vi "_setVariant.vi"(8 "error in (no error)":errorcluster, 9 "value":variant, 10 "name":string, 11 "DB Ref":T1) -> (0 "error in (no error) (dup)":errorcluster, 3 "DB Ref (dup)":T1, 4 "created?":bool)   [LabVIEW 2017, in "TagDB(dev).lvlib"]
uses:
  TagDB(dev).lvlib
  tagDB_Def.ctl
  <userlib>/_OpenG.lib/string/string.llb/Trim Whitespace (String)__ogtk.vi
  Error/_Build Error Cluster.vi
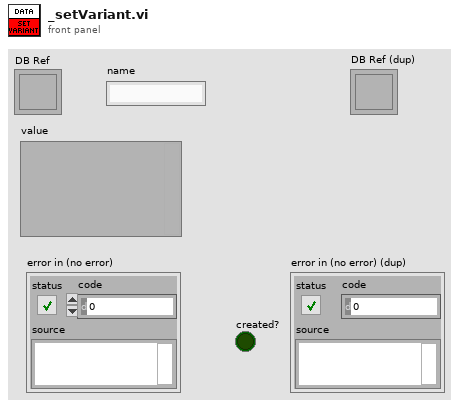
[diagram p1: front panel]
types:
  T1 = typedef "TagDB(dev).lvlib/tagDB_Def.ctl" = refnum<k1>
  T2 = typedef "TagDB(dev).lvlib/_DEF-DATA.ctl" = cluster{"data hashmap":variant, "DataChangeFlag":i64, "ItemChangeFlag":i64, "name":string, "Tag Adding Lock?":bool}
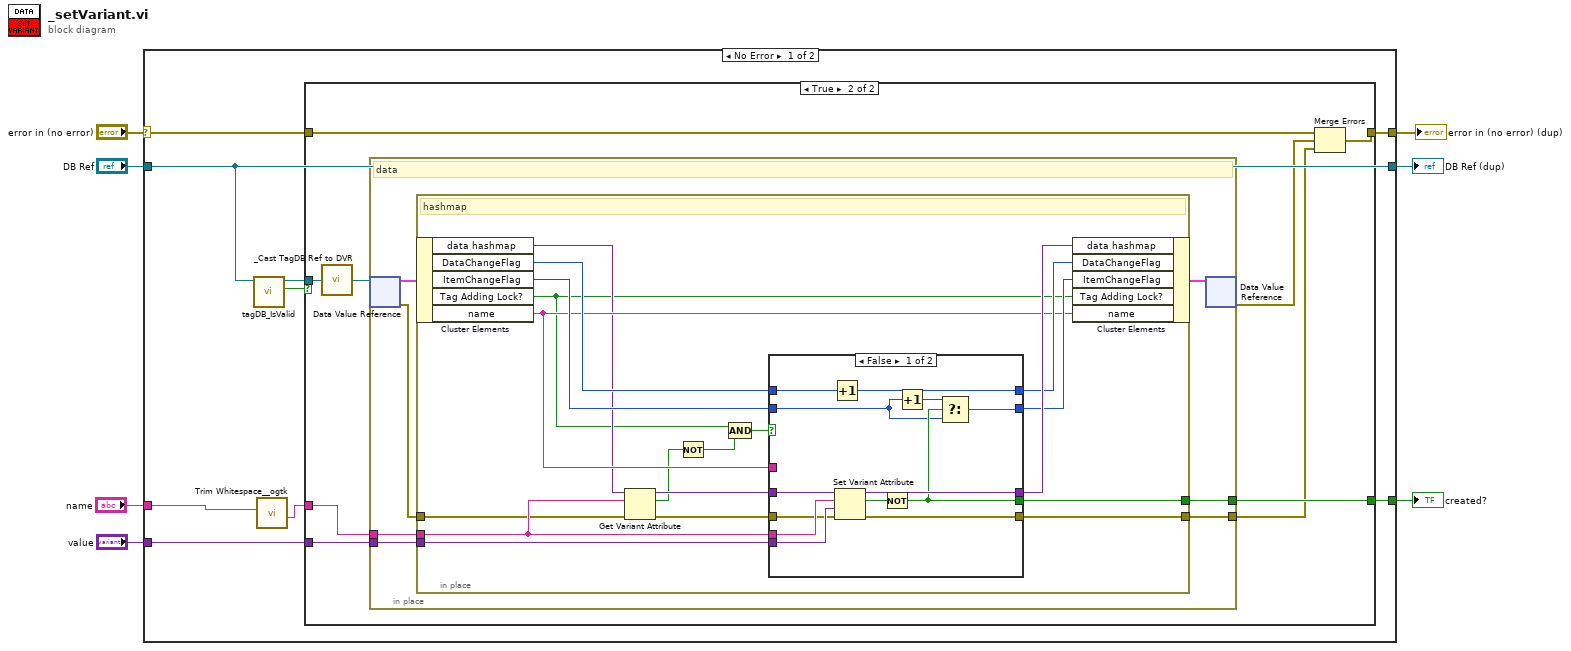
[diagram p0: block diagram]
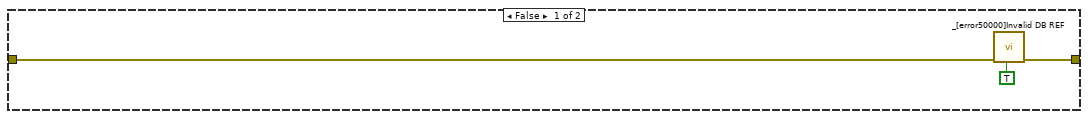
[diagram p2: hidden frame]
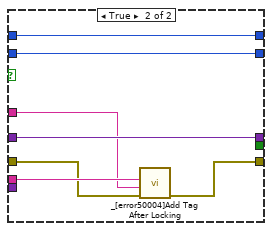
[diagram p3: hidden frame]
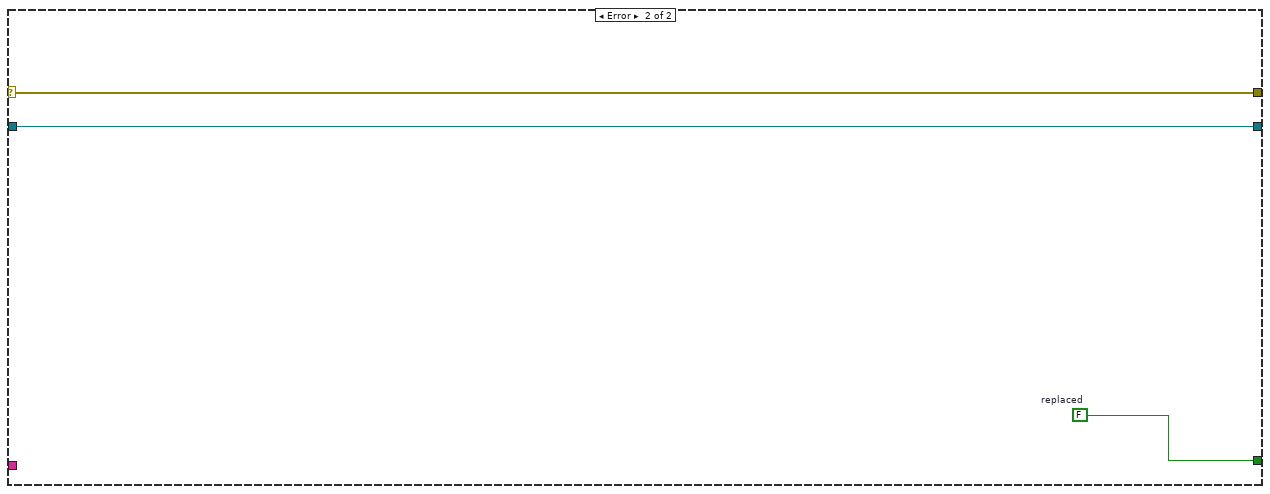
[diagram p4: hidden frame]
diagram:
  n1 = case shown="No Error" "error in (no error)" {
    selector: "error in (no error)" -> [w9 w75]
    tunnel: [w11 w76] -> w7
    tunnel: "DB Ref" -> [w11 w76]
    tunnel: [w15 w75] -> w4
    tunnel: [w16 w74] -> w3
    tunnel: "name" -> [w14 _]
    tunnel: "value" -> [w12 _]
    frame No Error {
      n2 = call "tagDB_IsValid.vi"("DB Ref in"=w11) -> ("valid?"=w8:bool, "DB Ref out"=w10:T1)  [unwired: 8 in, 1 out]
      n3 = call-poly <userlib>:"Trim Whitespace__ogtk.vi"("String in"=w14) -> ("String out"=w13:string)  [unwired: 6 in]
      n4 = case shown="True" w8 {
        tunnel: [_ w28] -> w16
        tunnel: [w18 w27] -> w15
        tunnel: w13 -> [_ w26]
        tunnel: w12 -> [_ w25]
        tunnel: w10 -> [_ w22]
        tunnel: w9 -> [w19 w21]
        frame False {
          n5 = call "_[error50000]Invalid DB REF.vi"("Force Gen?"=TRUE, "error in (no error)"=w19) -> ("error out"=w18:errorcluster)  [unwired: 9 in]
        }
        frame True {
          n6 = call "_Cast TagDB Ref to DVR.vi"("TagDB"=w22) -> ("DVR"=w23:refnum<data-value>)  [unwired: 4 in]
          n7 = in-place {
            in-place-border: [w33] -> w28
            in-place-border: w26 -> [w32]
            in-place-border: w25 -> [w31]
            in-place-border: [w30] -> w24
            # "data"
            n8 = in-place-dvr #1(w23) -> (w35:T2, w29:errorcluster)
            n9 = in-place {
              in-place-border: [w48] -> w33
              in-place-border: w32 -> [w38]
              in-place-border: w31 -> [w52]
              in-place-border: [w49] -> w30
              in-place-border: w29 -> [w36]
              # "hashmap"
              n10 = in-place-cluster #2(w35) -> ("data hashmap"=w44:variant, "DataChangeFlag"=w51:i64, "ItemChangeFlag"=w46:i64, "Tag Adding Lock?"=w40:bool, "name"=w45:string)
              n11 = Get Variant Attribute(Variant=w44, name=w38, error in=w36) -> (duplicate Variant=w43:variant, found=w41:bool, error out=w42:errorcluster)  [unwired: 1 in, 1 out]
              n12 = Not(x=w41) -> (.not. x?=w37:bool)
              n13 = Compound Arithmetic op=AND(w40, w37) -> (w39:bool)
              n14 = case shown="False" w39 {
                tunnel: w43 -> [w66 w73]
                tunnel: [w65 w73] -> w53
                tunnel: w38 -> [w63 w69]
                tunnel: w52 -> [w62 _]
                tunnel: w51 -> [w61 w72]
                tunnel: [w60 w72] -> w50
                tunnel: [w59 w70] -> w49
                tunnel: [w58 _] -> w48
                tunnel: [w57 w71] -> w47
                tunnel: w46 -> [w55 w71]
                tunnel: w45 -> [_ w68]
                tunnel: w42 -> [w54 w67]
                frame False {
                  n15 = Increment(x=w61) -> (x+1=w60:i64)
                  n16 = Set Variant Attribute(Variant=w66, name=w63, value=w62, error in=w54) -> (Variant out=w65:variant, replaced=w64:bool, error out=w59:errorcluster)
                  n17 = Not(x=w64) -> (.not. x?=w58:bool)
                  n18 = Increment(x=w55) -> (x+1=w56:i64)
                  n19 = Select(t=w56, s=w58, f=w55) -> (s? t:f=w57:i64)
                }
                frame True {
                  n20 = call "_[error50004]Add Tag After Locking.vi"("error in (no error)"=w67, "db name"=w68, "tag name"=w69) -> ("error out"=w70:errorcluster)  [unwired: 8 in]
                }
              }
              n21 = in-place-cluster #2("data hashmap"=w53, "DataChangeFlag"=w50, "ItemChangeFlag"=w47, "Tag Adding Lock?"=w40, "name"=w45) -> (w34:T2)
            }
            n22 = in-place-dvr #1(w34) -> (w20:errorcluster)  [unwired: 1 out]
          }
          n23 = Merge Errors(w21, w20, w24) -> (w27:errorcluster)
        }
      }
    }
    frame Error {
      w74 = FALSE  # replaced
    }
  }
  "DB Ref (dup)" <- w7
  "error in (no error) (dup)" <- w4
  "created?" <- w3
